vi "walletBalance_string.vi"(2 "String N":i32[](array[numeric]), 3 "Input String":string[](array[string])) -> (0 "Output String":string[](array[string]), 1 "after item 2":string[](array[string])=["SOL", "GST", "GMT", "USDC"])   [LabVIEW 2016]
panel:
  out "before item":string[](array[string])=["Run time & STEP", "Earn GST", "Energy", "Distance(km)", "Date time", "Shoe Type & Lv.", "Shoe #", "durability", "Δdura"]
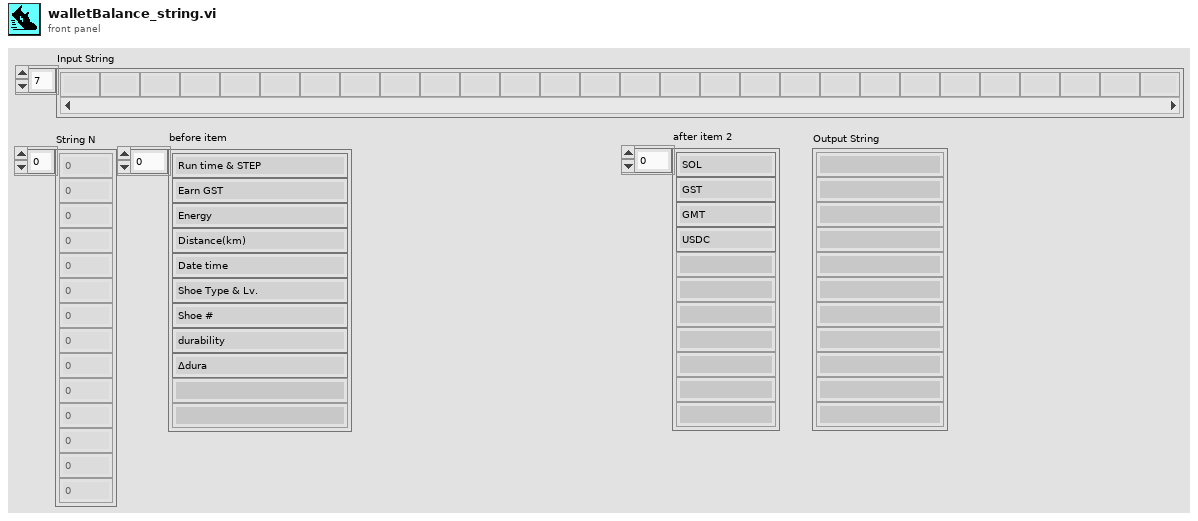
[diagram p1: front panel]
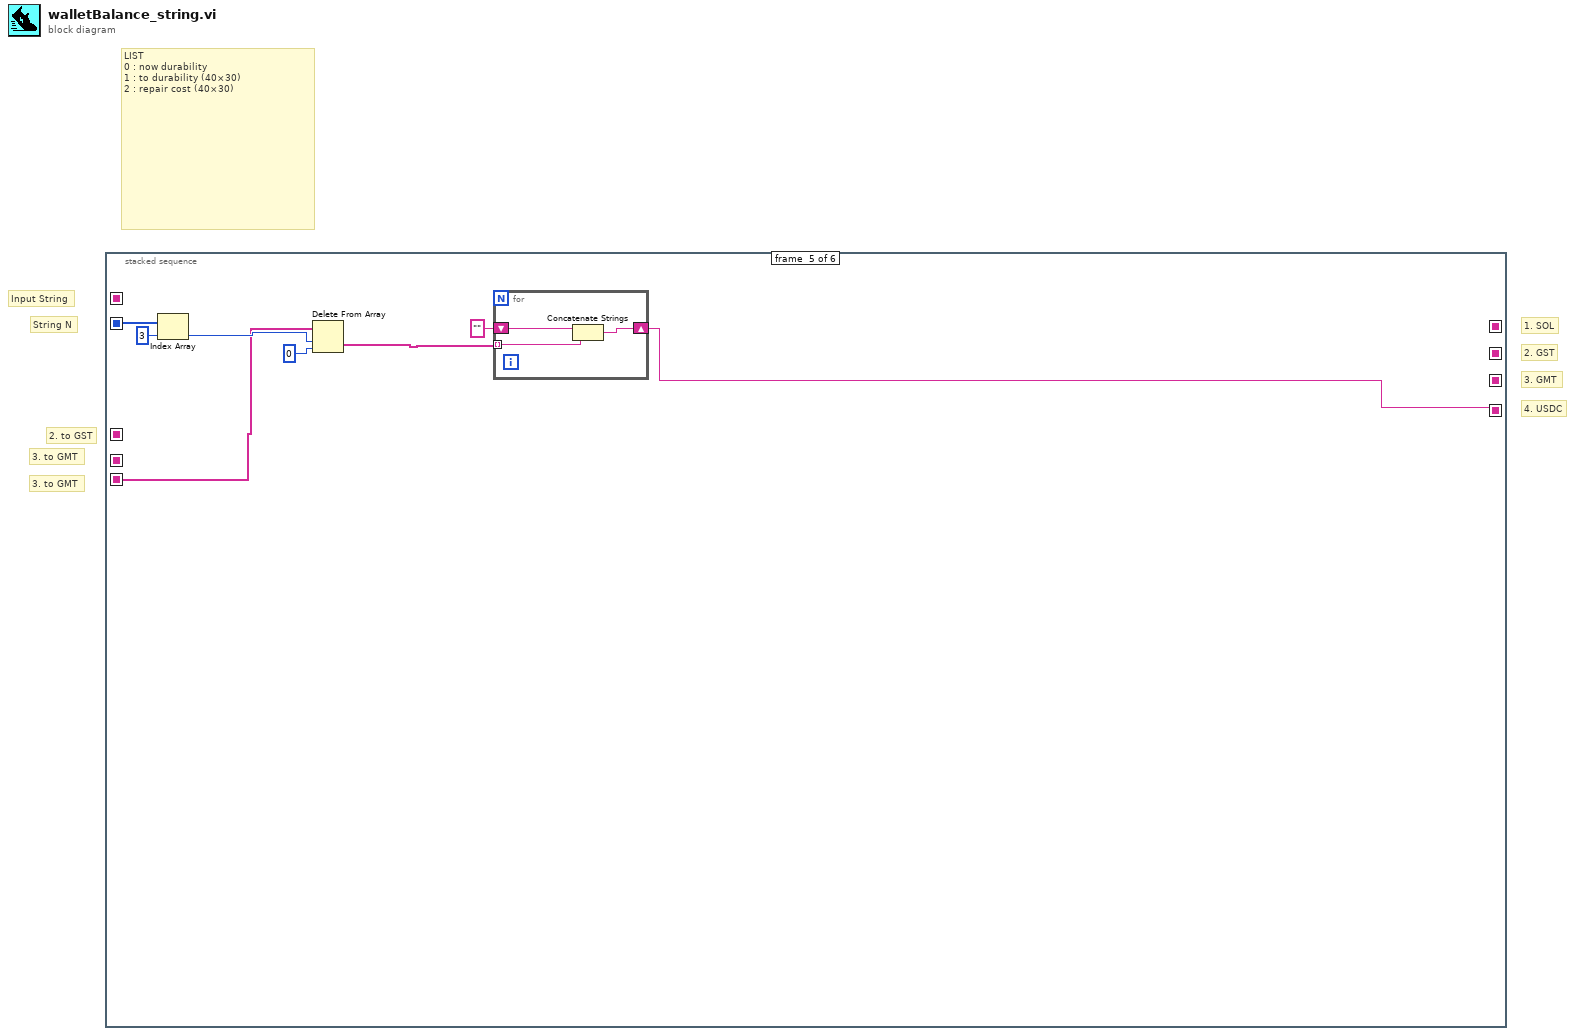
[diagram p0: block diagram]
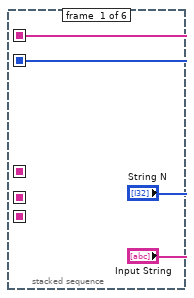
[diagram p2: hidden frame]
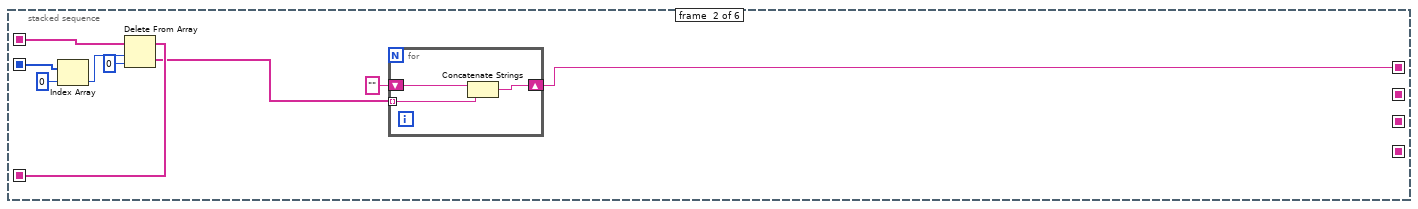
[diagram p3: hidden frame]
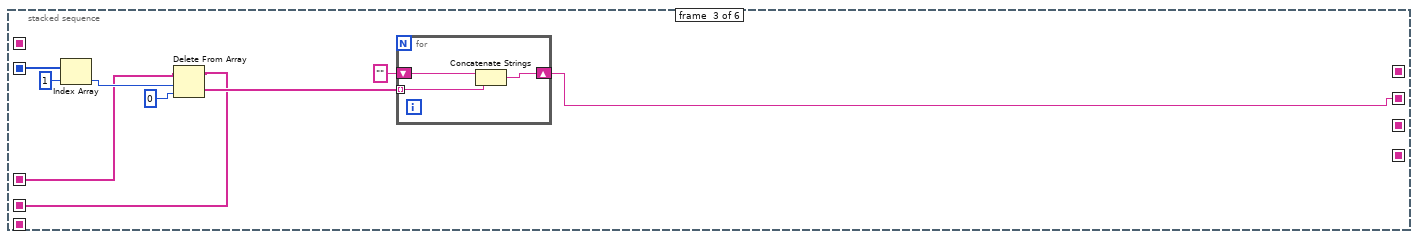
[diagram p4: hidden frame]
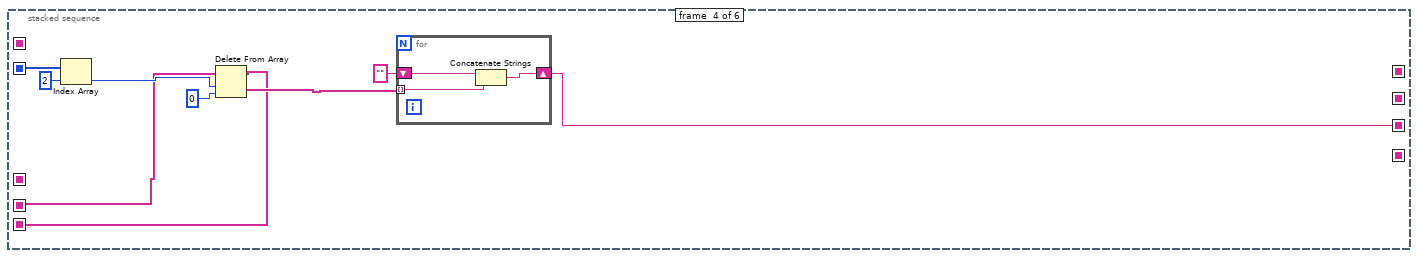
[diagram p5: hidden frame]
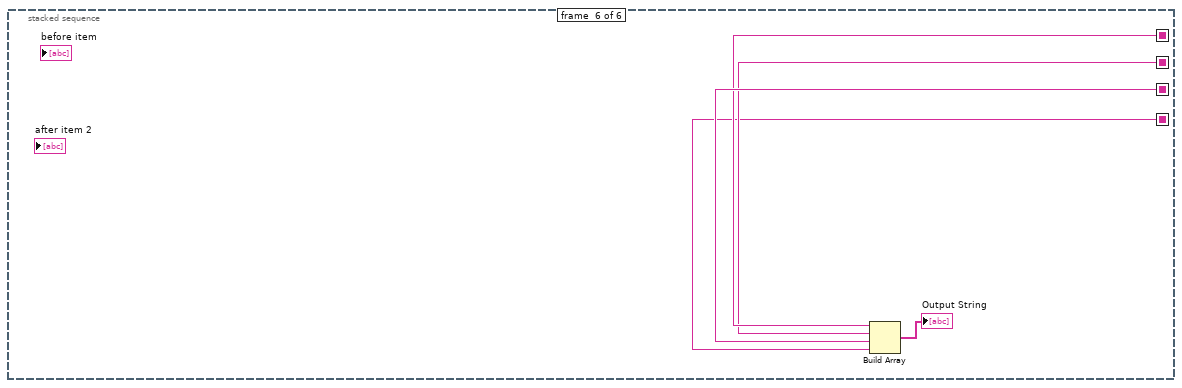
[diagram p6: hidden frame]
diagram:
  # "3. to GMT"
  # "4. USDC"
  # "3. to GMT"
  # "2. to GST"
  # "3. GMT"
  # "2. GST"
  # "1. SOL"
  # "LIST\n0 : now durability\n1 : to durability (40×30)\n2 : repair cost (40×30)"
  # "String N"
  # "Input String"
  n1 = stacked-sequence {
    seq-local: ["Input String" _ _ _ _ _] -> [_ w9 _ _ _ _]
    seq-local: ["String N" _ _ _ _ _] -> [_ w7 w19 w32 w43 _]
    seq-local: [_ w4 _ _ _ _] -> [_ _ w16 _ _ _]
    seq-local: [_ w10 _ _ _ _] -> [_ _ _ _ _ w52]
    seq-local: [_ _ w18 _ _ _] -> [_ _ _ _ _ w51]
    seq-local: [_ _ _ w31 _ _] -> [_ _ _ _ _ w53]
    seq-local: [_ _ w15 _ _ _] -> [_ _ _ w28 _ _]
    seq-local: [_ _ _ _ w39 _] -> [_ _ _ _ _ w50]
    seq-local: [_ _ _ w27 _ _] -> [_ _ _ _ w40 _]
    frame #0 {
    }
    frame #1 {
      n2 = Index Array(array=w7, index=0 ("指標")) -> (element=w6:i32)
      n3 = Delete From Array(array=w9, length=w6, index=0) -> (deleted portion=w3:string[], array with subset deleted=w4:string[])
      n4 = for {
        tunnel: w3 -> [w12] mode=indexing
        shift-right: [w14] -> w10
        shift-left: "" -> [w13]
        n5 = Concatenate Strings(w13, w12) -> (w14:string)
      }
    }
    frame #2 {
      n6 = Index Array(array=w19, index=1 ("指標")) -> (element=w17:i32)
      n7 = Delete From Array(array=w16, length=w17, index=0 ("指標")) -> (deleted portion=w20:string[], array with subset deleted=w15:string[])
      n8 = for {
        tunnel: w20 -> [w24] mode=indexing
        shift-right: [w26] -> w18
        shift-left: "" -> [w25]
        n9 = Concatenate Strings(w25, w24) -> (w26:string)
      }
    }
    frame #3 {
      n10 = Index Array(array=w32, index=2 ("指標")) -> (element=w30:i32)
      n11 = Delete From Array(array=w28, length=w30, index=0 ("指標")) -> (deleted portion=w29:string[], array with subset deleted=w27:string[])
      n12 = for {
        tunnel: w29 -> [w36] mode=indexing
        shift-right: [w38] -> w31
        shift-left: "" -> [w37]
        n13 = Concatenate Strings(w37, w36) -> (w38:string)
      }
    }
    frame #4 {
      n14 = Index Array(array=w43, index=3 ("指標")) -> (element=w42:i32)
      n15 = Delete From Array(array=w40, length=w42, index=0 ("指標")) -> (deleted portion=w41:string[])  [unwired: 1 out]
      n16 = for {
        tunnel: w41 -> [w47] mode=indexing
        shift-right: [w49] -> w39
        shift-left: "" -> [w48]
        n17 = Concatenate Strings(w48, w47) -> (w49:string)
      }
    }
    frame #5 {
      n18 = Build Array(w52, w51, w53, w50) -> (→"Output String":string[])
    }
  }
